vi "Configure Sweep Range Mode.vi"(8 "error in (no error)":errorcluster, 9 "Sweep Range Mode (2: Auto)":i32(ring)=2 items=["Best", "Fix", "Auto"], 10 "Channel (0: Channel 1)":i32(ring) items=["Channel 1", "Channel 2"], 11 "VISA resource name":refnum<visa-resource-name>) -> (0 "error out":errorcluster, 3 "VISA resource name out":refnum<visa-resource-name>)   [LabVIEW 2023, in "Agilent B2900 Series.lvlib"]
doc: "Configures sweep range mode for specified channel."
uses:
  Agilent B2900 Series.lvlib
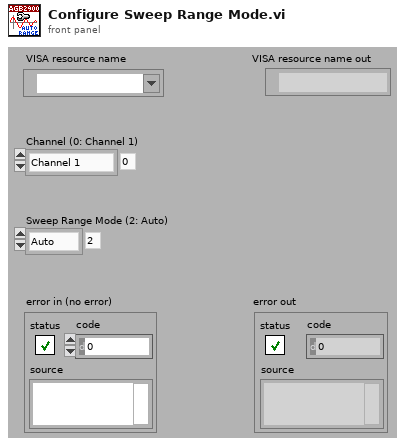
[diagram p1: front panel]
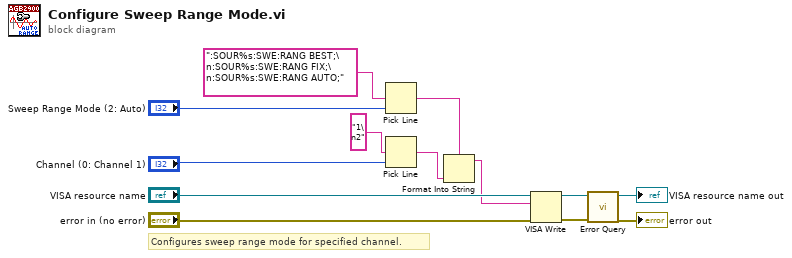
[diagram p0: block diagram]
diagram:
  # "Configures sweep range mode for specified channel."
  n1 = Pick Line(multi-line string=":SOUR%s:SWE:RANG BEST;\n:SOUR%s:SWE:RANG FIX;\n:SOUR%s:SWE:RANG AUTO;", line index="Sweep Range Mode (2: Auto)") -> (output string=w3:string)  [unwired: 1 in]
  n2 = Pick Line(multi-line string="1\n2" ("string (\"\")"), line index="Channel (0: Channel 1)") -> (output string=w1:string)  [unwired: 1 in]
  n3 = Format Into String(format string=w3, w1) -> (resulting string=w2:string)  [unwired: 2 in, 1 out]
  n4 = VISA Write(VISA resource name="VISA resource name", write buffer=w2, error in (no error)="error in (no error)") -> (VISA resource name out=w9:refnum<visa-resource-name>, error out=w8:errorcluster)  [unwired: 1 out]
  n5 = call "Error Query.vi"("error in (no error)"=w8, "VISA resource name"=w9) -> ("error out"=→"error out":errorcluster, "VISA resource name out"=→"VISA resource name out":refnum<visa-resource-name>)  [unwired: 6 in, 2 out]
